vi "decode_q11.vi"(6 "NumOfSignal":u8, 11 "Input Array u8":u8[](array[numeric]) format="%.0x") -> (3 "Output Plot":cluster{"X2":dbl[], "Y2":dbl[]}[](graph))   [LabVIEW 2020]
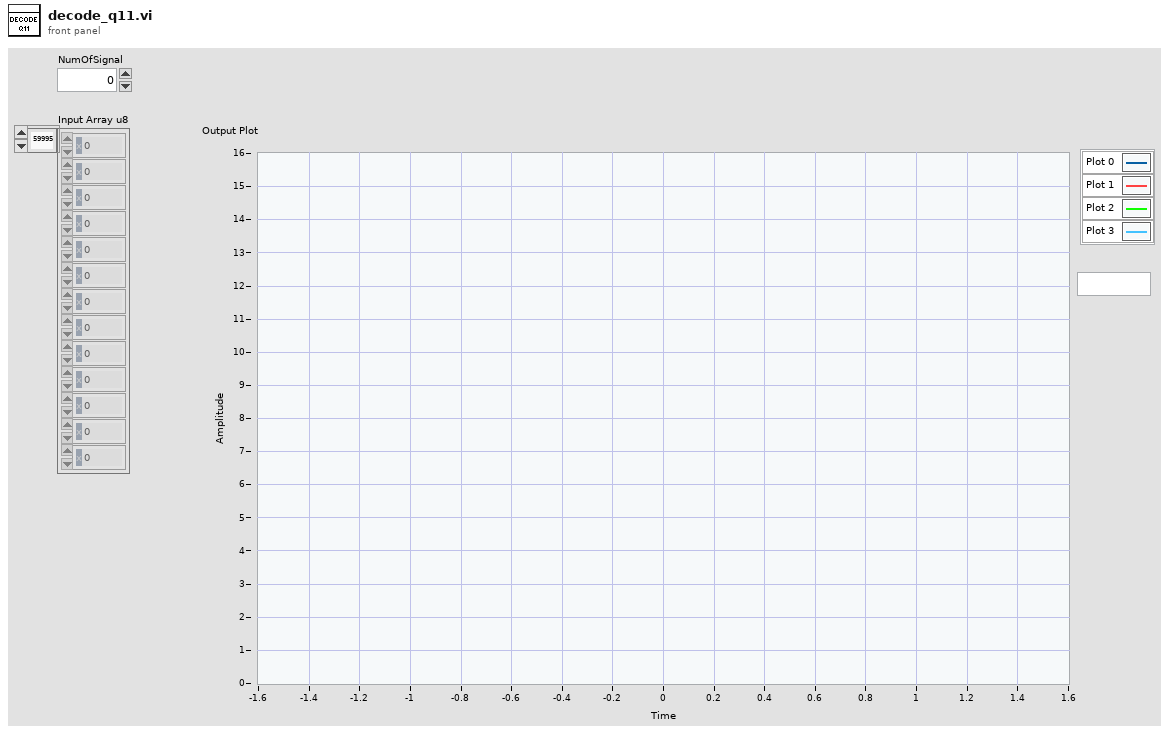
[diagram p1: front panel]
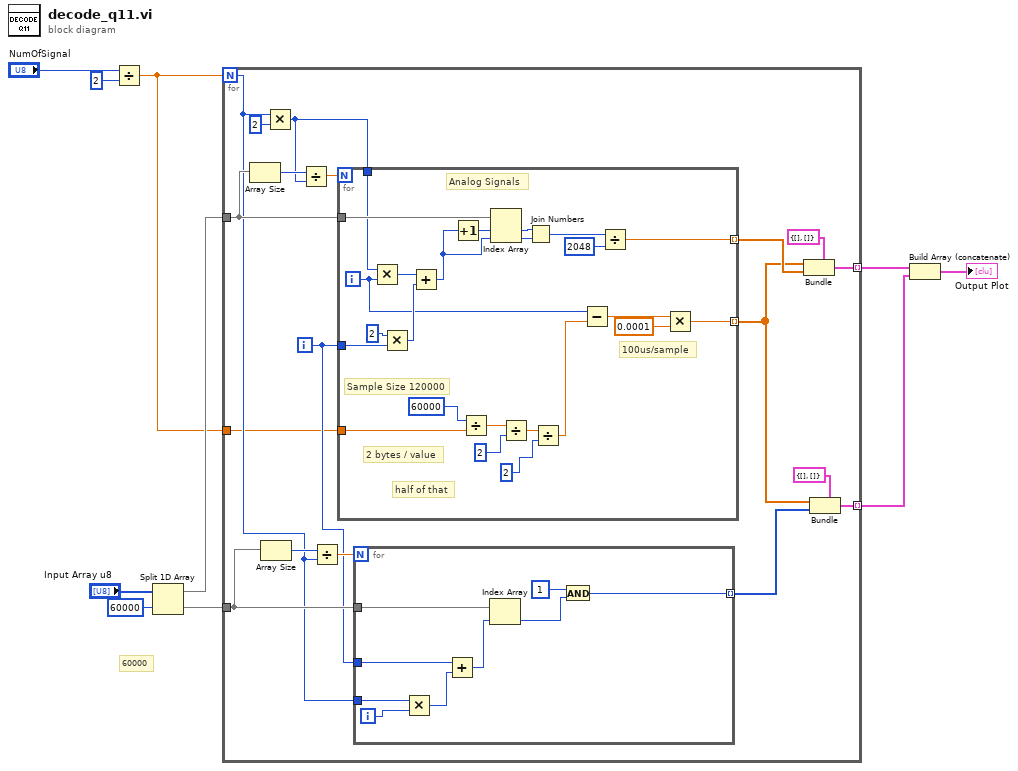
[diagram p0: block diagram]
diagram:
  # "60000"
  n1 = Divide(x="NumOfSignal", y=u8 2) -> (x/y=w1:dbl)
  n2 = Split 1D Array(array="Input Array u8", index=60000) -> (first subarray=w8:u8[], second subarray=w7:u8[])
  n3 = for {
    N: w1 -> [w15]
    tunnel: w8 -> [w26]
    tunnel: [w22] -> w6 mode=indexing
    tunnel: w7 -> [w18]
    tunnel: [w17] -> w5 mode=indexing
    tunnel: w1 -> [w11]
    i -> [w14]
    n4 = Array Size(array=w26) -> (size(s)=w28:i32)
    n5 = Array Size(array=w18) -> (size(s)=w20:i32)
    n6 = Multiply(x=w15, y=2) -> (x*y=w24:i32)
    n7 = Divide(x=w28, y=w24) -> (x/y=w27:dbl)
    n8 = Divide(x=w20, y=w15) -> (x/y=w19:dbl)
    n9 = for {
      N: w27 -> [_]
      tunnel: w26 -> [w61]
      tunnel: w24 -> [w57]
      tunnel: w14 -> [w56]
      tunnel: [w49] -> w21 mode=indexing
      tunnel: [w40] -> w13 mode=indexing
      tunnel: w11 -> [w38]
      i -> [w48]
      # "Analog Signals"
      # "100us/sample"
      # "half of that"
      # "2 bytes / value"
      # "Sample Size 120000"
      n10 = Multiply(x=w57, y=w48) -> (x*y=w53:i32)
      n11 = Multiply(x=2 ("y"), y=w56) -> (x*y=w54:i32)
      n12 = Add(x=w53, y=w54) -> (x+y=w52:i32)
      n13 = Increment(x=w52) -> (x+1=w58:i32)
      n14 = Divide(x=60000, y=w38) -> (x/y=w46:dbl)
      n15 = Index Array(array=w61, index #1=w58, index #2=w52) -> (element #1=w60:u8, element #2=w59:u8)
      n16 = Divide(x=w46, y=2 ("x")) -> (x/y=w44:dbl)
      n17 = Join Numbers(hi=w60, lo=w59) -> ((hi.lo)=w50:u16)
      n18 = Divide(x=w44, y=2 ("x")) -> (x/y=w42:dbl)
      n19 = Subtract(x=w48, y=w42) -> (x-y=w41:dbl)
      n20 = Divide(x=w50, y=2048 ("x")) -> (x/y=w49:dbl)
      n21 = Multiply(x=w41, y=0.0001) -> (x*y=w40:dbl)
    }
    n22 = for {
      N: w19 -> [_]
      tunnel: w18 -> [w32]
      tunnel: w15 -> [w36]
      tunnel: w14 -> [w34]
      tunnel: [w29] -> w12 mode=indexing
      i -> [w37]
      n23 = Multiply(x=w36, y=w37) -> (x*y=w35:i32)
      n24 = Add(x=w34, y=w35) -> (x+y=w33:i32)
      n25 = Index Array(array=w32, index=w33) -> (element=w31:u8)
      n26 = And(x=u8 1, y=w31) -> (x .and. y?=w29:u8)
    }
    n27 = Bundle(cluster=cluster{"X1":dbl[], "Y1":dbl[]} {"X1"=[], "Y1"=[]} ("output cluster"), "X1"=w13, "Y1"=w21) -> (w22:cluster{"X1":dbl[], "Y1":dbl[]})
    n28 = Bundle(cluster=cluster{"X1":dbl[], "Y1":dbl[]} {"X1"=[], "Y1"=[]} ("output cluster"), "X1"=w13, "Y1"=w12) -> (w17:cluster{"X1":dbl[], "Y1":dbl[]})
  }
  n29 = Build Array (concatenate)(w6, w5) -> (→"Output Plot":cluster{"X1":dbl[], "Y1":dbl[]}[])
